vi "Get LV Glyph Path.vi"(7 "Path":T1, 8 "error in (no error)":errorcluster, 11 "File Name":string) -> (0 "error out":errorcluster, 3 "Requested Path":path)   [LabVIEW 2020, in "lv_icon.lvlib"]
doc: "Get the path to the palettes for Glyphs and Templates."
uses:
  resource/plugins/lv_icon.lvlib
  Controls/Pathes.ctl
panel:
  in  "VI":string="VI"
  in  "Library":string="Library"
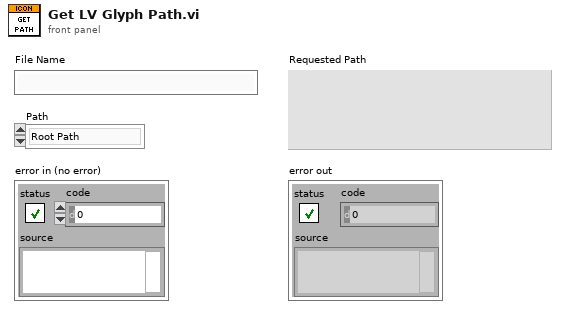
[diagram p1: front panel]
types:
  T1 = typedef "Pathes.ctl" = enum16{"Root Path", "Icon Templates", "Icon Templates VI", "Icon Templates Lib", "Glyphs"}
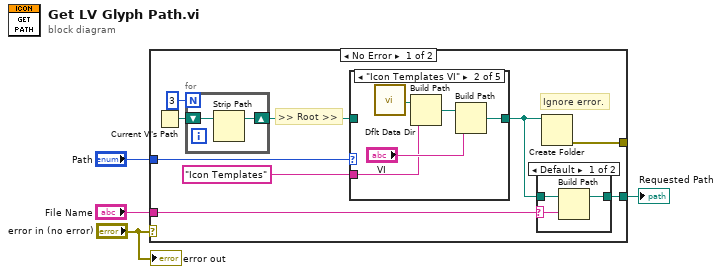
[diagram p0: block diagram]
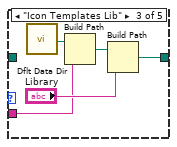
[diagram p4: hidden frame]
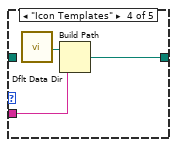
[diagram p5: hidden frame]
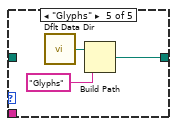
[diagram p6: hidden frame]
diagram:
  n1 = case shown="No Error" "error in (no error)" {
    tunnel: "File Name" -> [w6 _]
    tunnel: "Path" -> [w13 _]
    tunnel: [w9 _] -> w1
    tunnel: [w5 _] -> _
    frame No Error {
      # "Ignore error."
      # ">> Root >>"
      n2 = Current VI's Path() -> (path=w12:path)
      n3 = for {
        N: 3 -> [_]
        shift-right: [w18] -> w10
        shift-left: w12 -> [w19]
        n4 = Strip Path(path=w19) -> (stripped path=w18:path)  [unwired: 1 out]
      }
      n5 = case shown="\"Icon Templates VI\"" w13 {
        tunnel: w10 -> [w20 _ _ _ _]
        tunnel: [w20 w22 w27 w32 w34] -> w8
        tunnel: "Icon Templates" ("Icon Templates") -> [_ w21 w26 w31 _]
        frame "Root Path", Default {
        }
        frame "Icon Templates VI" {
          n6 = call <vilib>:"Dflt Data Dir.vi"() -> ("App:Default Data Directory"=w25:path)
          n7 = Build Path(base path=w25, name or relative path=w21) -> (appended path=w24:path)
          n8 = Build Path(base path=w24, name or relative path="VI") -> (appended path=w22:path)
        }
        frame "Icon Templates Lib" {
          n9 = call <vilib>:"Dflt Data Dir.vi"() -> ("App:Default Data Directory"=w30:path)
          n10 = Build Path(base path=w30, name or relative path=w26) -> (appended path=w29:path)
          n11 = Build Path(base path=w29, name or relative path="Library") -> (appended path=w27:path)
        }
        frame "Icon Templates" {
          n12 = call <vilib>:"Dflt Data Dir.vi"() -> ("App:Default Data Directory"=w33:path)
          n13 = Build Path(base path=w33, name or relative path=w31) -> (appended path=w32:path)
        }
        frame "Glyphs" {
          n14 = call <vilib>:"Dflt Data Dir.vi"() -> ("App:Default Data Directory"=w35:path)
          n15 = Build Path(base path=w35, name or relative path="Glyphs" ("Glyphs")) -> (appended path=w34:path)
        }
      }
      n16 = case shown="Default" w6 {
        selector: w6 -> [w14 _]
        tunnel: w8 -> [w16 w17]
        tunnel: [w15 w17] -> w9
        frame Default {
          n17 = Build Path(base path=w16, name or relative path=w14) -> (appended path=w15:path)
        }
        frame "" {
        }
      }
      n18 = Create Folder(path (use dialog)=w8) -> (error out=w5:errorcluster)  [unwired: 1 in, 3 out]
    }
    frame Error {
    }
  }
  "Requested Path" <- w1
  "error out" <- "error in (no error)"
